vi "Read IntegrationTime.vi"(8 "error in (no error)":errorcluster, 11 "ElectrometerInternalConfiguration in":refnum<class "ElectrometerInternalConfiguration.lvclass">) -> (0 "error out":errorcluster, 2 "IntegrationTime":dbl=0.002, 3 "ElectrometerInternalConfiguration out":refnum<class "ElectrometerInternalConfiguration.lvclass">)   [LabVIEW 2016, in "ElectrometerInternalConfiguration.lvclass"]
uses:
  ElectrometerInternalConfiguration.lvclass
  ElectrometerInternalConfiguration.lvclass/ElectrometerInternalConfiguration.ctl
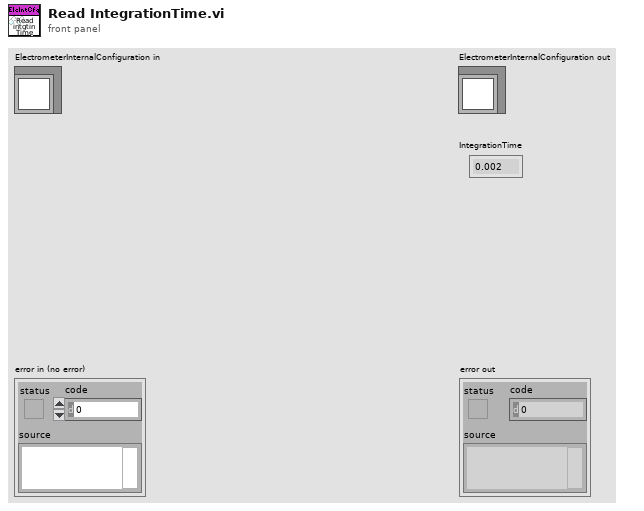
[diagram p1: front panel]
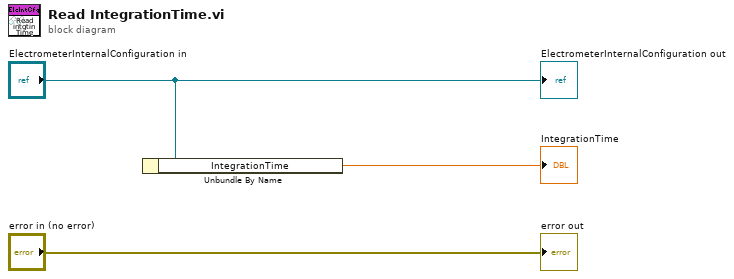
[diagram p0: block diagram]
diagram:
  n1 = Unbundle By Name("ElectrometerInternalConfiguration in") -> ("IntegrationTime"=→"IntegrationTime":dbl)
  "error out" <- "error in (no error)"
  "ElectrometerInternalConfiguration out" <- "ElectrometerInternalConfiguration in"
